vi "Get Pattern.vi"(11 "Section File Interface":refnum<class "Section File Interface.lvclass">) -> (2 "file extension":string)   [LabVIEW 2020, in "ImportExport.lvlib" / "Section File Interface.lvclass"]
uses:
  Section File Interface.lvclass
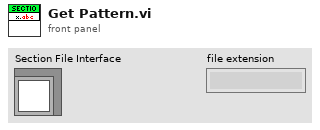
[diagram p1: front panel]
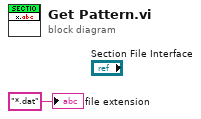
[diagram p0: block diagram]
diagram:
  "file extension" <- "*.dat" ("file extension")
